vi "MetaData Parameters FG.vi"(7 "Action":T1, 8 "error in (no error)":errorcluster, 10 "MetaData Parameters":T3={"Data Type"=enum."Single Channel", "Channel Type"=enum."Format", "List"=[], "Format String"="%.3g", "Type"=enum."SGL", "Delimiter"=",", "Endian"=enum."Native"}, 11 "Item Ref in":T2 format="%.0x") -> (0 "error out":errorcluster, 2 "MetaData Parameters":T3={"Data Type"=enum."Single Channel", "Channel Type"=enum."Format", "List"=[], "Format String"="%.3g", "Type"=enum."SGL", "Delimiter"=",", "Endian"=enum."Native"}, 3 "Item Ref out":T2 format="%.0x")   [LabVIEW 2020, in "Instrument Addon Shared.lvlib"]
uses:
  Instrument Addon Shared.lvlib
  MetaData Parameters.ctl
  Protocol Data Type.ctl
  Metadata Channel Type.ctl
  Type Cast Type.ctl
  Endian.ctl
  <vilib>/NI VeriStand/Custom Device API/Custom Device Item Ref.ctl
  FG Control.ctl
  Constants.vi
  <vilib>/NI VeriStand/Custom Device API/Get Item Property (U32).vi
  <vilib>/NI VeriStand/Custom Device API/Get Item Property (String Array).vi
  <vilib>/NI VeriStand/Custom Device API/Get Item Property (String).vi
  <vilib>/NI VeriStand/Custom Device API/Set Item Property (U32).vi
  <vilib>/NI VeriStand/Custom Device API/Set Item Property (String Array).vi
  <vilib>/NI VeriStand/Custom Device API/Set Item Property (String).vi
  <vilib>/NI VeriStand/Custom Device API/Custom Device API.lvlib
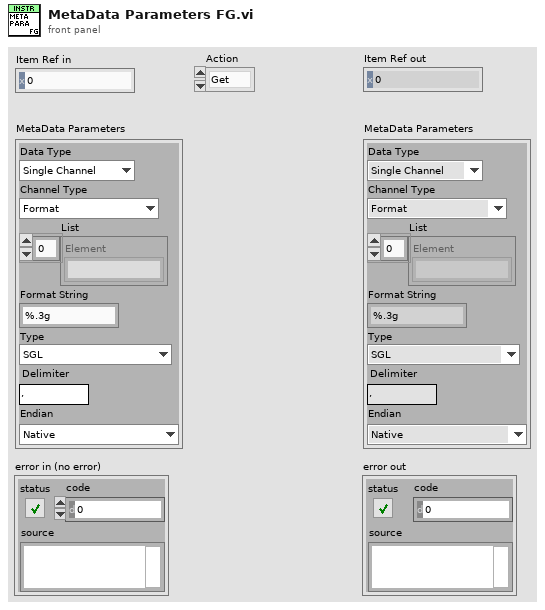
[diagram p1: front panel]
types:
  T1 = typedef "Instrument Addon Shared.lvlib/FG Control.ctl" = enum16{"Get", "Set"}
  T2 = typedef "Custom Device API.lvlib/Custom Device Item Ref.ctl" = u64
  T3 = typedef "Instrument Addon Shared.lvlib/MetaData Parameters.ctl" = cluster{"Data Type":T4, "Channel Type":T5, "List":string[], "Format String":string, "Type":T6, "Delimiter":string, "Endian":T7}
  T4 = typedef "Instrument Addon Shared.lvlib/Protocol Data Type.ctl" = enum16{"Single Channel", "Array"}
  T5 = typedef "Instrument Addon Shared.lvlib/Metadata Channel Type.ctl" = enum16{"Enumerated List", "Format", "Type Cast"}
  T6 = typedef "Instrument Addon Shared.lvlib/Type Cast Type.ctl" = enum16{"DBL", "SGL", "U64", "U32", "U16", "U8", "I64", "I32", "I16", "I8"}
  T7 = typedef "Instrument Addon Shared.lvlib/Endian.ctl" = enum16{"Native", "Little", "Big"}
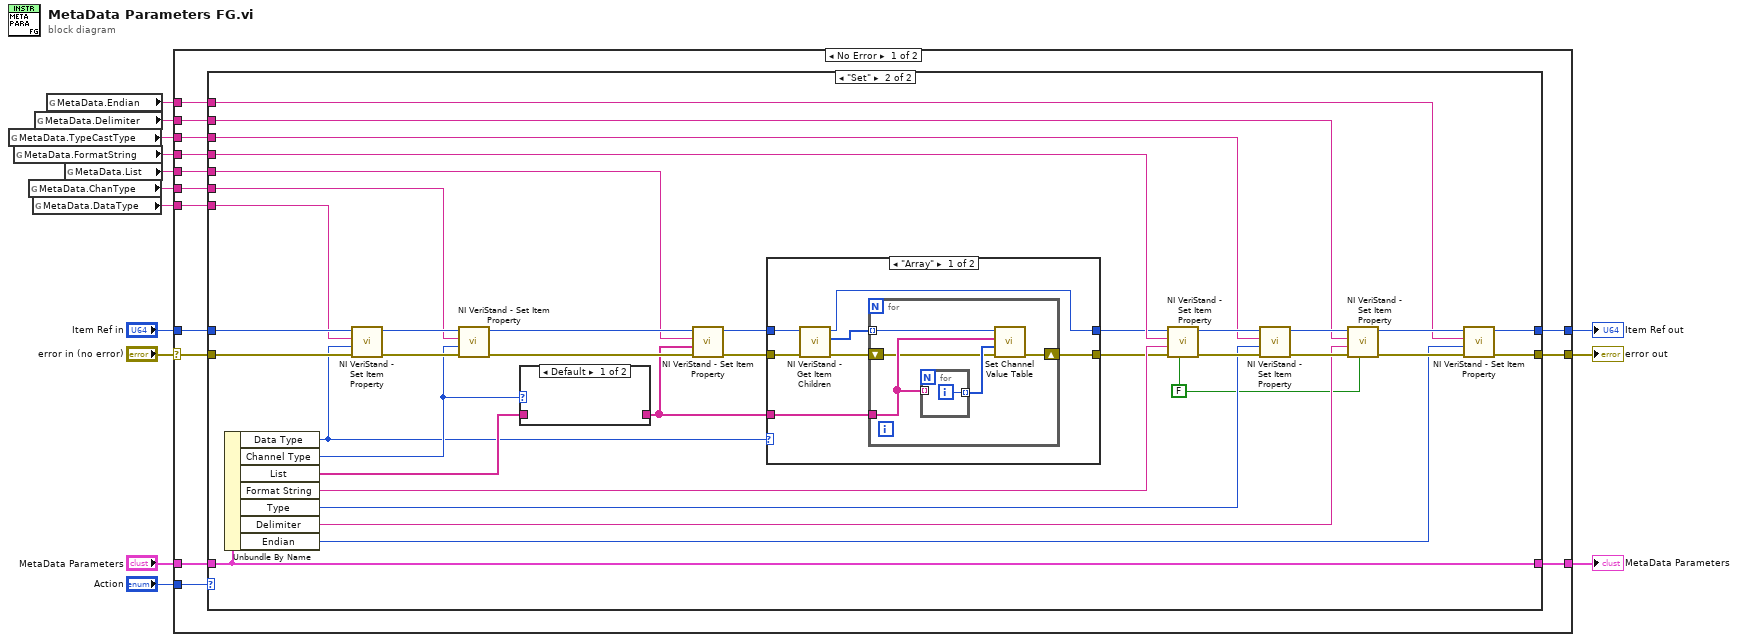
[diagram p0: block diagram]
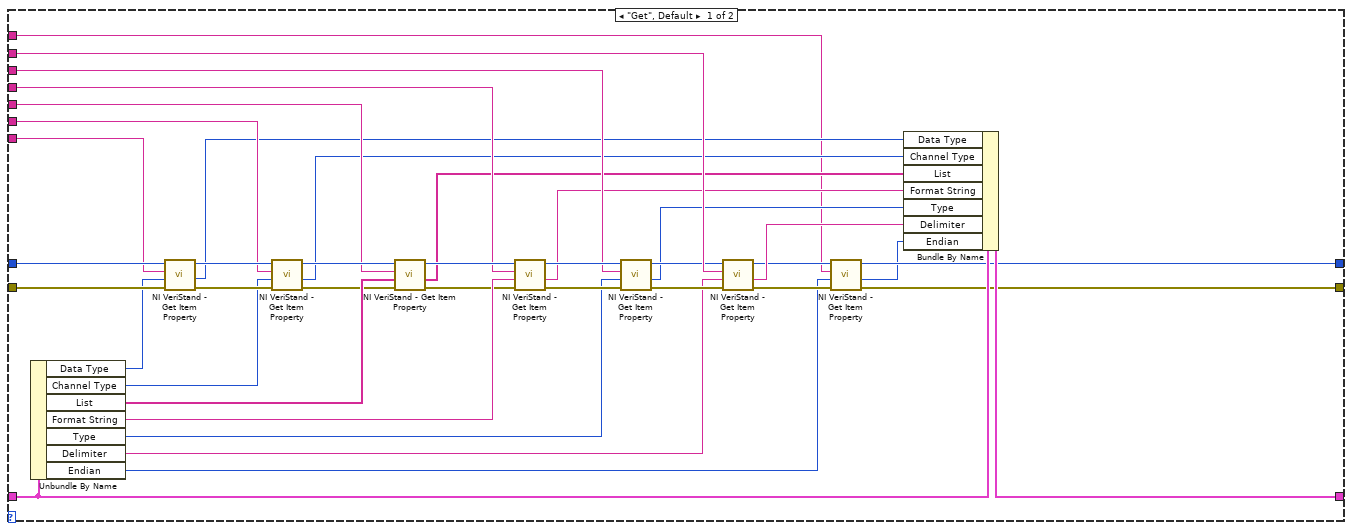
[diagram p2: hidden frame]
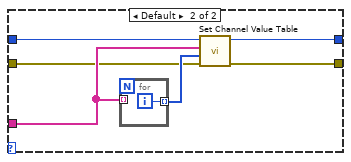
[diagram p3: hidden frame]
diagram:
  n1 = global read "Constants.vi" "MetaData.TypeCastType"() -> (w2:string)
  n2 = global read "Constants.vi" "MetaData.FormatString"() -> (w3:string)
  n3 = global read "Constants.vi" "MetaData.ChanType"() -> (w5:string)
  n4 = global read "Constants.vi" "MetaData.DataType"() -> (w6:string)
  n5 = global read "Constants.vi" "MetaData.Delimiter"() -> (w8:string)
  n6 = global read "Constants.vi" "MetaData.Endian"() -> (w1:string)
  n7 = global read "Constants.vi" "MetaData.List"() -> (w4:string)
  n8 = case shown="No Error" "error in (no error)" {
    selector: "error in (no error)" -> [w23 w126]
    tunnel: w8 -> [w28 _]
    tunnel: [w27 w124] -> w12
    tunnel: "Item Ref in" -> [w26 w124]
    tunnel: "MetaData Parameters" -> [w25 w125]
    tunnel: [w24 w126] -> w11
    tunnel: [w22 w125] -> w7
    tunnel: "Action" -> [w21 _]
    tunnel: w6 -> [w20 _]
    tunnel: w5 -> [w19 _]
    tunnel: w4 -> [w18 _]
    tunnel: w3 -> [w17 _]
    tunnel: w2 -> [w16 _]
    tunnel: w1 -> [w15 _]
    frame No Error {
      n9 = case shown="\"Set\"" w21 {
        tunnel: w28 -> [w47 w82]
        tunnel: [w34 w78] -> w27
        tunnel: w26 -> [w66 w102]
        tunnel: w25 -> [w43 w99]
        tunnel: [w32 w80] -> w24
        tunnel: w23 -> [w67 w101]
        tunnel: [w36 w99] -> w22
        tunnel: w20 -> [w62 w100]
        tunnel: w19 -> [w61 w86]
        tunnel: w18 -> [w56 w85]
        tunnel: w17 -> [w52 w84]
        tunnel: w16 -> [w48 w83]
        tunnel: w15 -> [w31 w76]
        frame "Get", Default {
          n10 = Unbundle By Name(w43) -> ("Data Type"=w65:T4, "Channel Type"=w60:T5, "List"=w59:string[], "Format String"=w55:string, "Type"=w49:T6, "Delimiter"=w44:string, "Endian"=w30:T7)
          n11 = call-poly <vilib>:"NI VeriStand - Get Item Property.vi"("error in (no error)"=w67, "Default Value"=w65, "Property Name"=w62, "Item Ref in"=w66) -> ("error out"=w64:errorcluster, "Value"=w37:u32, "Item Ref out"=w63:T2)  [unwired: 4 in, 1 out]
          n12 = call-poly <vilib>:"NI VeriStand - Get Item Property.vi"("error in (no error)"=w64, "Default Value"=w60, "Property Name"=w61, "Item Ref in"=w63) -> ("error out"=w58:errorcluster, "Value"=w38:u32, "Item Ref out"=w57:T2)  [unwired: 4 in, 1 out]
          n13 = call-poly <vilib>:"NI VeriStand - Get Item Property.vi"("error in (no error)"=w58, "Default Value"=w59, "Property Name"=w56, "Item Ref in"=w57) -> ("error out"=w54:errorcluster, "Value"=w39:string[], "Item Ref out"=w53:T2)  [unwired: 4 in, 1 out]
          n14 = call-poly <vilib>:"NI VeriStand - Get Item Property.vi"("error in (no error)"=w54, "Default Value"=w55, "Property Name"=w52, "Item Ref in"=w53) -> ("error out"=w51:errorcluster, "Value"=w40:string, "Item Ref out"=w50:T2)  [unwired: 4 in, 1 out]
          n15 = call-poly <vilib>:"NI VeriStand - Get Item Property.vi"("error in (no error)"=w51, "Default Value"=w49, "Property Name"=w48, "Item Ref in"=w50) -> ("error out"=w45:errorcluster, "Value"=w41:u32, "Item Ref out"=w46:T2)  [unwired: 4 in, 1 out]
          n16 = call-poly <vilib>:"NI VeriStand - Get Item Property.vi"("error in (no error)"=w45, "Default Value"=w44, "Property Name"=w47, "Item Ref in"=w46) -> ("error out"=w33:errorcluster, "Value"=w42:string, "Item Ref out"=w35:T2)  [unwired: 4 in, 1 out]
          n17 = call-poly <vilib>:"NI VeriStand - Get Item Property.vi"("error in (no error)"=w33, "Default Value"=w30, "Property Name"=w31, "Item Ref in"=w35) -> ("error out"=w32:errorcluster, "Value"=w29:u32, "Item Ref out"=w34:T2)  [unwired: 4 in, 1 out]
          n18 = Bundle By Name(cluster=w43, "Data Type"=w37, "Channel Type"=w38, "List"=w39, "Format String"=w40, "Type"=w41, "Delimiter"=w42, "Endian"=w29) -> (w36:T3)
        }
        frame "Set" {
          w87 = FALSE ("Binary String (T)")
          n19 = Unbundle By Name(w99) -> ("Data Type"=w68:T4, "Channel Type"=w71:T5, "List"=w70:string[], "Format String"=w90:string, "Type"=w89:T6, "Delimiter"=w88:string, "Endian"=w77:T7)
          n20 = call-poly <vilib>:"NI VeriStand - Set Item Property.vi"("error in (no error)"=w101, "Value"=w68, "Property Name"=w100, "Item Ref in"=w102) -> ("error out"=w91:errorcluster, "Item Ref out"=w98:T2)  [unwired: 5 in, 1 out]
          n21 = call-poly <vilib>:"NI VeriStand - Set Item Property.vi"("error in (no error)"=w91, "Value"=w71, "Property Name"=w86, "Item Ref in"=w98) -> ("error out"=w92:errorcluster, "Item Ref out"=w97:T2)  [unwired: 5 in, 1 out]
          n22 = case shown="Default" w71 {
            tunnel: w70 -> [_ w123]
            tunnel: [_ w123] -> w69
            frame Default {
            }
            frame "Enumerated List" {
            }
          }
          n23 = call-poly <vilib>:"NI VeriStand - Set Item Property.vi"("error in (no error)"=w92, "Value"=w69, "Property Name"=w85, "Item Ref in"=w97) -> ("error out"=w75:errorcluster, "Item Ref out"=w73:T2)  [unwired: 5 in, 1 out]
          n24 = case shown="\"Array\"" w68 {
            tunnel: w75 -> [w106 w118]
            tunnel: [w109 w116] -> w74
            tunnel: w73 -> [w107 w120]
            tunnel: [w103 w117] -> w72
            tunnel: w69 -> [w108 w119]
            frame "Array" {
              n25 = call <vilib>:"NI VeriStand - Get Item Children.vi"("error in (no error)"=w106, "Item Ref in"=w107) -> ("error out"=w105:errorcluster, "Child Refs"=w104:T2[], "Item Ref out"=w103:T2)  [unwired: 6 in, 1 out]
              n26 = for {
                tunnel: w108 -> [w113]
                tunnel: w104 -> [w114] mode=indexing
                shift-right: [w110] -> w109
                shift-left: w105 -> [w111]
                n27 = for {
                  tunnel: w113 -> [_] mode=indexing
                  tunnel: [w115] -> w112 mode=indexing
                  i -> [w115]
                }
                n28 = call "Set Channel Value Table.vi"("Error In"=w111, "Values"=w112, "Names"=w113, "Channel Ref In"=w114) -> ("Error Out"=w110:errorcluster)  [unwired: 6 in, 1 out]
              }
            }
            frame Default {
              n29 = for {
                tunnel: w119 -> [_] mode=indexing
                tunnel: [w122] -> w121 mode=indexing
                i -> [w122]
              }
              n30 = call "Set Channel Value Table.vi"("Error In"=w118, "Values"=w121, "Names"=w119, "Channel Ref In"=w120) -> ("Error Out"=w116:errorcluster, "Channel Ref Out"=w117:T2)  [unwired: 6 in]
            }
          }
          n31 = call-poly <vilib>:"NI VeriStand - Set Item Property.vi"("Binary String (T)"=w87, "error in (no error)"=w74, "Value"=w90, "Property Name"=w84, "Item Ref in"=w72) -> ("error out"=w93:errorcluster, "Item Ref out"=w96:T2)  [unwired: 4 in, 1 out]
          n32 = call-poly <vilib>:"NI VeriStand - Set Item Property.vi"("error in (no error)"=w93, "Value"=w89, "Property Name"=w83, "Item Ref in"=w96) -> ("error out"=w94:errorcluster, "Item Ref out"=w95:T2)  [unwired: 5 in, 1 out]
          n33 = call-poly <vilib>:"NI VeriStand - Set Item Property.vi"("Binary String (T)"=w87, "error in (no error)"=w94, "Value"=w88, "Property Name"=w82, "Item Ref in"=w95) -> ("error out"=w81:errorcluster, "Item Ref out"=w79:T2)  [unwired: 4 in, 1 out]
          n34 = call-poly <vilib>:"NI VeriStand - Set Item Property.vi"("error in (no error)"=w81, "Value"=w77, "Property Name"=w76, "Item Ref in"=w79) -> ("error out"=w80:errorcluster, "Item Ref out"=w78:T2)  [unwired: 5 in, 1 out]
        }
      }
    }
    frame Error {
    }
  }
  "error out" <- w11
  "MetaData Parameters" <- w7
  "Item Ref out" <- w12
